vi "719 Initial Tree.vi"(8 "error in (no error)":errorcluster caption="错误输入（无错误）", 11 "树形控件":refnum<vi>) -> (0 "error out":errorcluster caption="错误输出")   [LabVIEW 2018]
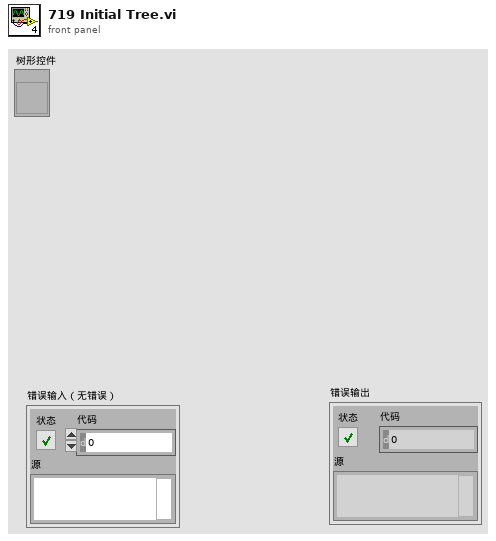
[diagram p1: front panel]
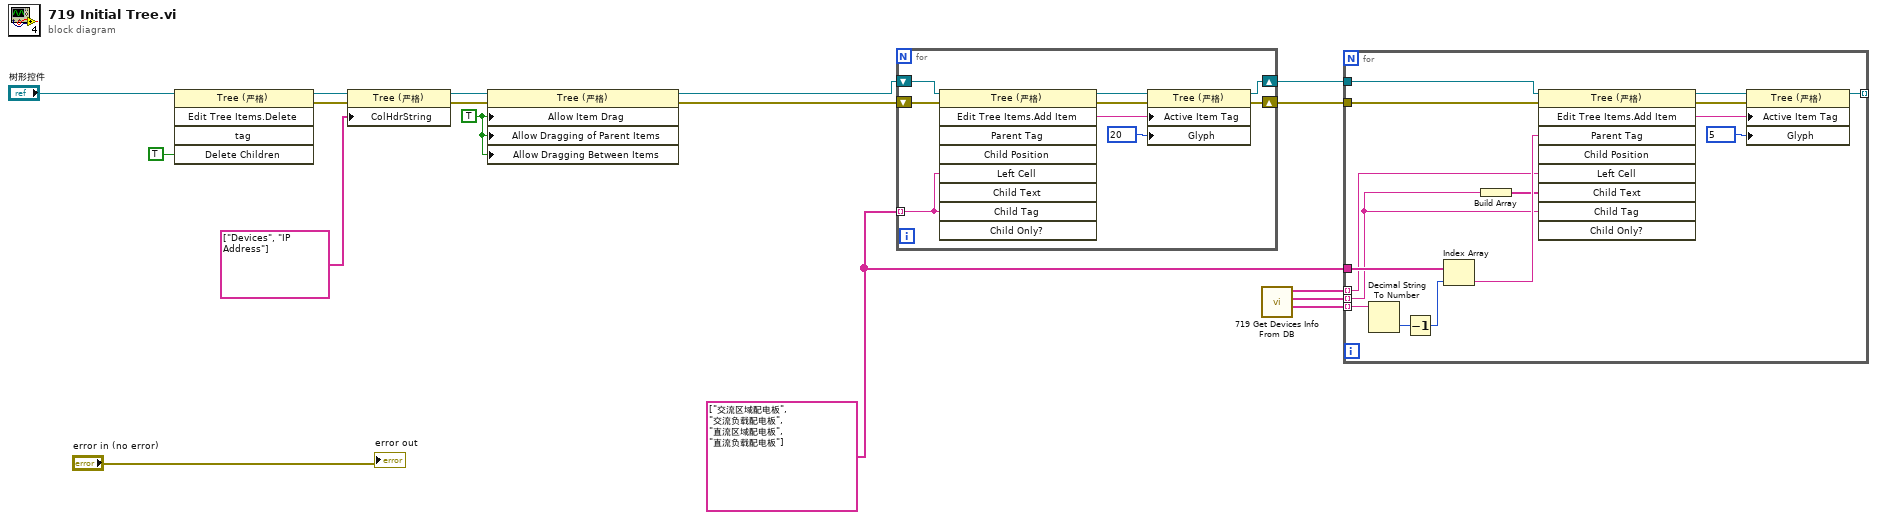
[diagram p0: block diagram]
diagram:
  w6 = string[] ["交流区域配电板", "交流负载配电板", "直流区域配电板", "直流负载配电板"] ("左单元格字符串")
  w15 = TRUE ("拖曳/放置:允许拖曳")
  n1 = invoke class="Tree (严格)" method="Edit Tree Items.Delete"(reference="树形控件", "Delete Children"=TRUE ("删除子项？")) -> (reference out=w7:refnum<vi>, error out=w13:errorcluster)  [unwired: 3 in, 3 out]
  n2 = property class="Tree (严格)"(reference=w7, error in=w13, "ColHdrString"=string[] ["Devices", "IP Address"] ("列首字符串[]")) -> (reference out=w14:refnum<vi>, error out=w12:errorcluster)
  n3 = property class="Tree (严格)"(reference=w14, error in=w12, "Allow Item Drag"=w15, "Allow Dragging of Parent Items"=w15, "Allow Dragging Between Items"=w15) -> (reference out=w11:refnum<vi>, error out=w10:errorcluster)
  n4 = for {
    tunnel: w6 -> [w18] mode=indexing
    shift-right: [w20] -> w9
    shift-left: w11 -> [w26]
    shift-right: [w19] -> w8
    shift-left: w10 -> [w25]
    n5 = invoke class="Tree (严格)" method="Edit Tree Items.Add Item"(reference=w26, error in=w25, "Left Cell"=w18, "Child Tag"=w18) -> (reference out=w24:refnum<vi>, error out=w23:errorcluster, "Edit Tree Items:Add Item"=w22:string)  [unwired: 5 in, 6 out]
    n6 = property class="Tree (严格)"(reference=w24, error in=w23, "Active Item Tag"=w22, "Glyph"=20) -> (reference out=w20:refnum<vi>, error out=w19:errorcluster)
  }
  n7 = call "719 Get Devices Info From DB.vi"() -> ("Type"=w1:string[], "IP Address"=w3:string[], "Device Name"=w2:string[])  [unwired: 8 in, 1 out]
  n8 = for {
    tunnel: w9 -> [w37]
    tunnel: w8 -> [w36]
    tunnel: [w35] -> _ mode=indexing
    tunnel: w6 -> [w32]
    tunnel: w2 -> [w28] mode=indexing
    tunnel: w3 -> [w27] mode=indexing
    tunnel: w1 -> [w34] mode=indexing
    n9 = Decimal String To Number(string=w34) -> (number=w33:i32)  [unwired: 2 in, 1 out]
    n10 = Decrement(x=w33) -> (x-1=w31:i32)
    n11 = Index Array(array=w32, index=w31) -> (element=w30:string)
    n12 = Build Array(w27) -> (w29:string[])
    n13 = invoke class="Tree (严格)" method="Edit Tree Items.Add Item"(reference=w37, error in=w36, "Parent Tag"=w30, "Left Cell"=w28, "Child Text"=w29, "Child Tag"=w27) -> (reference out=w38:refnum<vi>, error out=w39:errorcluster, "Edit Tree Items:Add Item"=w40:string)  [unwired: 3 in, 6 out]
    n14 = property class="Tree (严格)"(reference=w38, error in=w39, "Active Item Tag"=w40, "Glyph"=5) -> (reference out=w35:refnum<vi>)  [unwired: 1 out]
  }
  "error out" <- "error in (no error)"
